vi "PolFlag_LocalControl.vi"(4 "error in (no error)":errorcluster) -> (0 "error out":errorcluster, 1 "Paired = 1":i32, 2 "Switch Verify Sense":string, 3 "Position (0=open, 1=closed)":i32)   [LabVIEW 2009]
doc: "Local control of polarization flag sent to receiver"
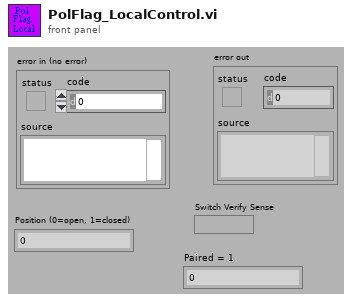
[diagram p1: front panel]
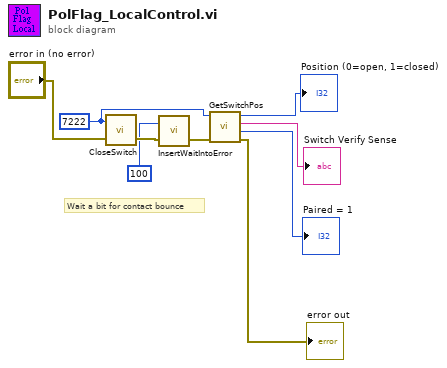
[diagram p0: block diagram]
diagram:
  w8 = 7222
  # "Wait a bit for contact bounce"
  n1 = call "CloseSwitch.vi"("error in (no error)"="error in (no error)", "Switch ID"=w8) -> ("error out"=w6:errorcluster)  [unwired: 1 in]
  n2 = call "InsertWaitIntoError.vi"("error in (no error)"=w6, "Wait (msecs)"=100) -> ("error out"=w5:errorcluster)  [unwired: 1 in]
  n3 = call "GetSwitchPos.vi"("error in (no error)"=w5, "Circuit ID"=w8) -> ("Error out"=→"error out":errorcluster, "Paired = 1"=→"Paired = 1":i32, "Switch Position Verify  Sense"=→"Switch Verify Sense":string, "Position (0=open, 1=closed)"=→"Position (0=open, 1=closed)":i32)  [unwired: 2 in]
